vi "Panel.vi"(11 "ControlBindingPanel in":refnum<class "ControlBindingPanel.lvclass">) -> ()   [LabVIEW 2020, in "VolatusGUIEditor.lvlib" / "ControlBindingPanel.lvclass"]
uses:
  ControlBindingPanel.lvclass
  C:/dev/lv20CE/relink/lv-oopanel/OOPanel/Panel/Panel.lvclass
  lv-oopanel/OOPanel/Panel/Basic UI State.ctl
  ControlBindingPanel.lvclass/ControlBindingPanel.ctl
  Control Bind Data.ctl
  lv-tree-tools/Tree Map/Tree Map/Tree Map.lvclass
  lv-oopanel/OOPanel/Panel/Panel.lvclass
  lv-oopanel/OOPanel/OOPanel.lvlib
  VolatusGUIEditor.lvlib
panel:
  in  "Select":bool
  in  "Tree":string(tree)
  # "Selected element is not bound to a control type.\nSet the control type from the list below:"
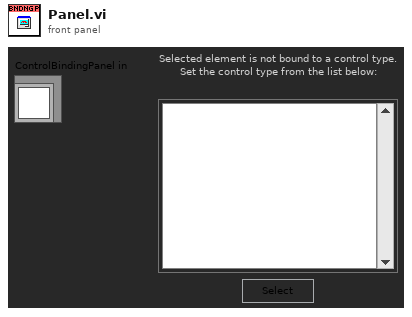
[diagram p1: front panel]
types:
  T1 = typedef "OOPanel.lvlib/Panel.lvclass/Basic UI State.ctl" = enum16{"Init", "Run", "Close"}
  T2 = enum8{"Enabled", "Disabled", "Disabled and Grayed Out"}
  T3 = typedef "VolatusGUIEditor.lvlib/Control Bind Data.ctl" = cluster{"Ctl Refnum":refnum<vi>, "Type Name":string}
  T4 = typedef "VolatusGUIEditor.lvlib/ControlBindingPanel.lvclass/Incoming Events.ctl" = cluster{"Update Control":refnum<user-event>, "Update Tree":refnum<user-event>}
  T5 = typedef "OOPanel.lvlib/Panel.lvclass/Panel Events.ctl" = cluster{"Visbility":refnum<user-event>, "Close":refnum<user-event>}
  T6 = typedef "OOPanel.lvlib/Visibility State.ctl" = enum16{"Idle", "Closed", "Hidden", "Visible", "Subpanel", "Hidden Subpanel"}
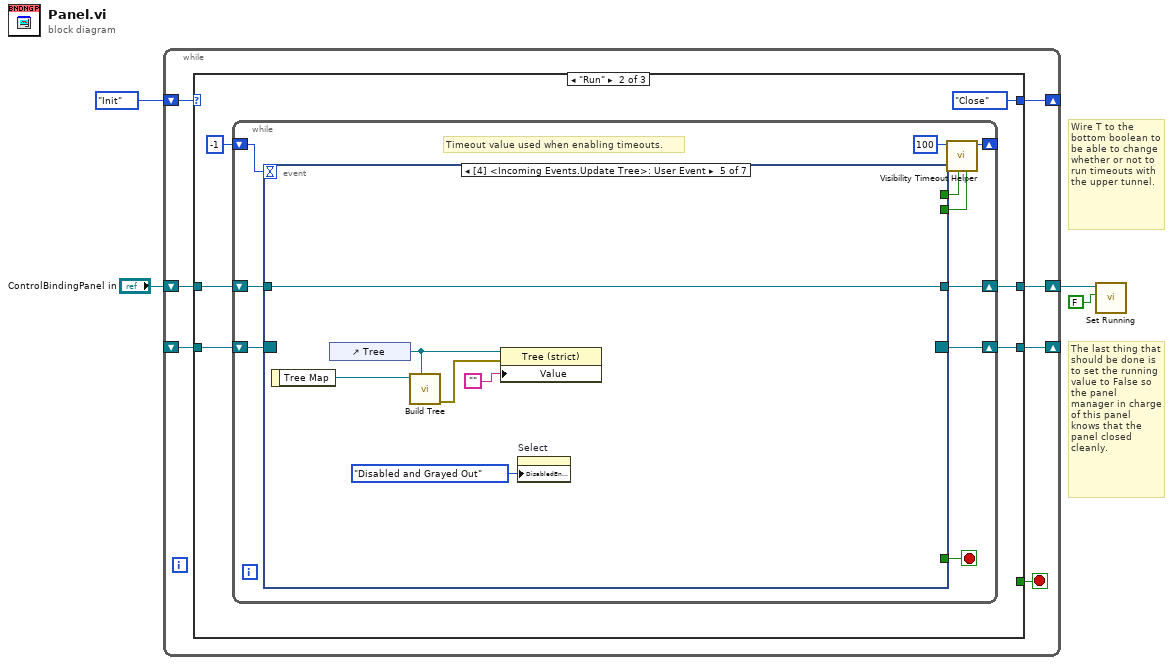
[diagram p0: block diagram]
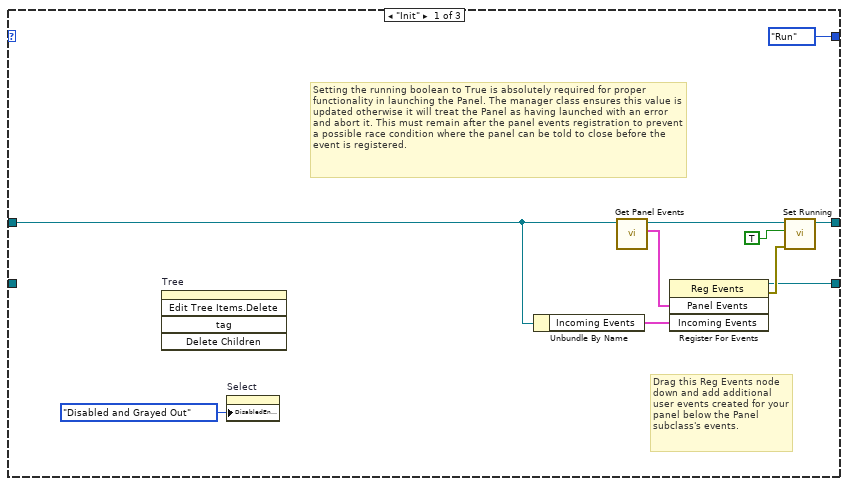
[diagram p2: hidden frame]
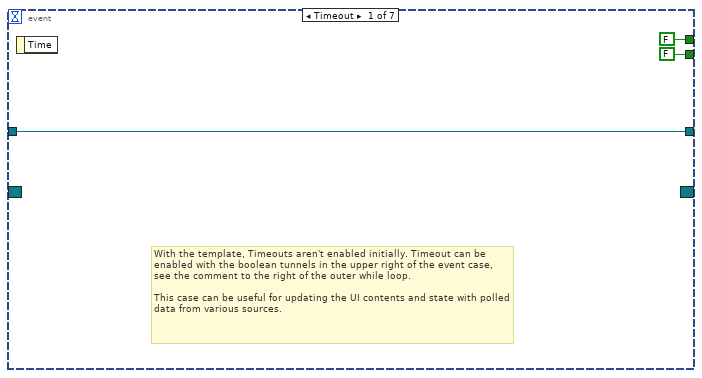
[diagram p3: hidden frame]
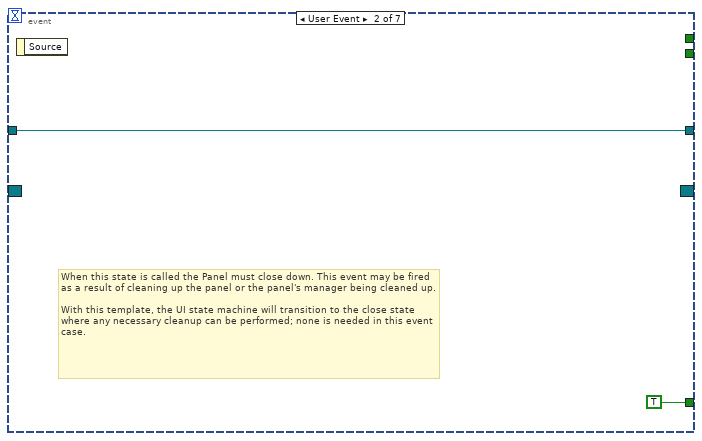
[diagram p4: hidden frame]
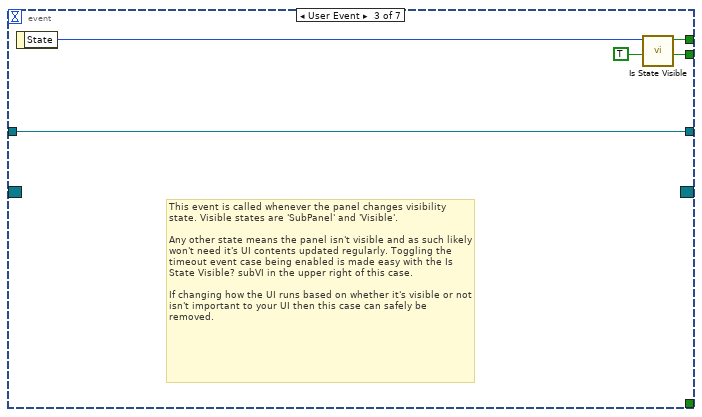
[diagram p5: hidden frame]
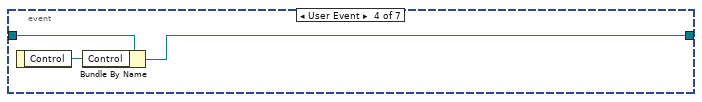
[diagram p6: hidden frame]
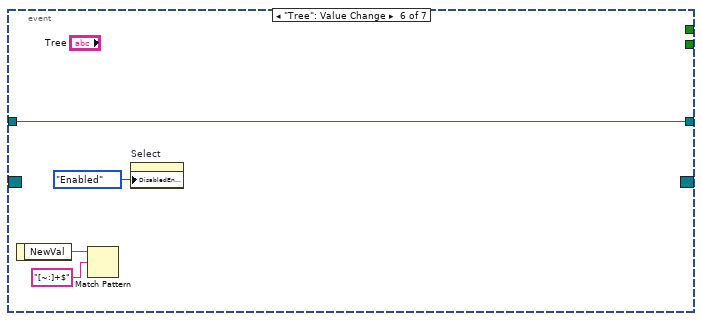
[diagram p7: hidden frame]
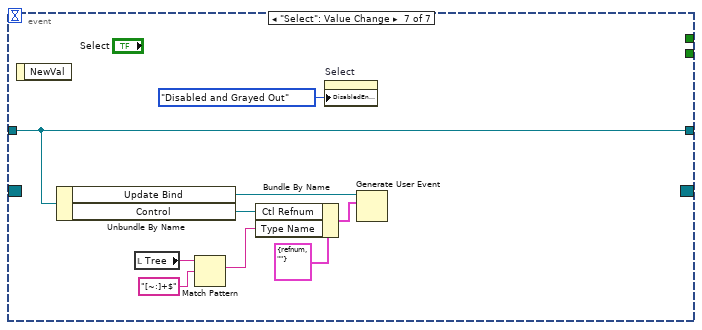
[diagram p8: hidden frame]
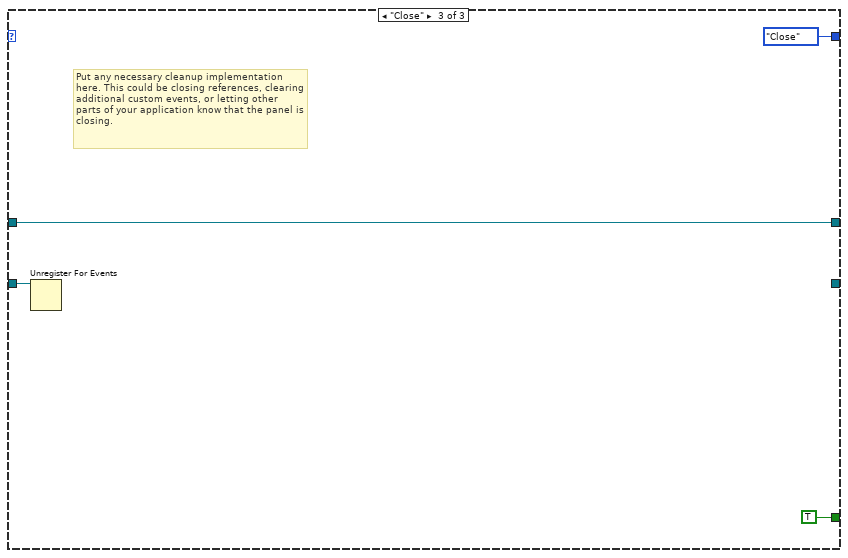
[diagram p9: hidden frame]
diagram:
  # "The last thing that should be done is to set the running value to False so the panel manager in charge of this panel knows that the panel closed cleanly."
  # "Wire T to the bottom boolean to be able to change whether or not to run timeouts with the upper tunnel."
  n1 = while {
    shift-right: [w10] -> _
    shift-left: _ -> [w11]
    shift-right: [w8] -> _
    shift-left: Basic_UI_State."Init" ("Basic UI State") -> [w9]
    shift-right: [w6] -> w4
    shift-left: "ControlBindingPanel in" -> [w5]
    stop <- w7 stop-if-true
    n2 = case shown="\"Run\"" w9 {
      tunnel: w11 -> [_ w27 w70]
      tunnel: [w18 w25 _] -> w10
      tunnel: [Basic_UI_State."Run" ("Basic UI State") Basic_UI_State."Close" ("Basic UI State") Basic_UI_State."Close" ("Basic UI State")] -> w8
      tunnel: [_ _ TRUE] -> w7
      tunnel: [w17 w22 w69] -> w6
      tunnel: w5 -> [w13 w23 w69]
      frame "Init" {
        # "Setting the running boolean to True is absolutely required for proper functionality in launching the Panel. The manager class ensures this value is updated otherwise it will treat the Panel as having launched with an error and abort it. This must remain after the panel events registration to prevent a possible race condition where the panel can be told to close before the event is registered."
        # "Drag this Reg Events node down and add additional user events created for your panel below the Panel subclass's events."
        n3 = invoke on="Tree" class="Tree (strict)" method="Edit Tree Items.Delete"() -> ()  [unwired: 5 in, 5 out]
        n4 = property on="Select" class="Bool"("DisabledEnum"=T2."Disabled and Grayed Out" ("Disabled")) -> ()  [unwired: 2 in, 2 out]
        n5 = Unbundle By Name(w13) -> ("Incoming Events"=w12:T4)
        n6 = call "Get Panel Events.vi"("Panel in"=w13) -> ("Panel Events"=w15:T5, "Panel out"=w16:refnum<class "ControlBindingPanel.lvclass">)  [unwired: 8 in, 1 out]
        n7 = register-events(w15, w12) -> (reference out=w18:refnum<event-registration>, error out=w20:errorcluster)  [unwired: 2 in]
        n8 = call "Set Running.vi"("error in (no error)"=w20, "Running"=TRUE, "Panel in"=w16) -> ("Panel out"=w17:refnum<class "ControlBindingPanel.lvclass">)  [unwired: 7 in, 1 out]
      }
      frame "Run" {
        n9 = while {
          shift-right: [w33] -> w25
          shift-left: w27 -> [w34]
          shift-right: [w36] -> _
          shift-left: -1 ("Timeout") -> [w35]
          shift-right: [w28] -> w22
          shift-left: w23 -> [w29]
          stop <- w30 stop-if-true
          # "Timeout value used when enabling timeouts."
          n10 = event shown="[4] <Incoming Events.Update Tree>: User Event" {
            selector: w34 -> [_ _ _ _ _ _ _]
            dyn-events: [_ _ _ _ _ _ _] -> w33
            timeout: w35 -> [_ _ _ _ _ _ _]
            tunnel: [FALSE _ w45 _ _ _ _] -> w32
            tunnel: [FALSE _ TRUE _ _ _ _] -> w31
            tunnel: [_ TRUE _ _ _ _ _] -> w30
            tunnel: w29 -> [w38 w41 w43 w49 w55 w59 w66]
            tunnel: [w38 w41 w43 w48 w55 w59 w66] -> w28
            event Timeout {
              # "With the template, Timeouts aren't enabled initially. Timeout can be enabled with the boolean tunnels in the upper right of the event case, see the comment to the right of the outer while loop.\n\nThis case can be useful for updating the UI contents and state with polled data from various sources."
              n11 = event-data() -> ()  [unwired: 1 in, 1 out]
            }
            event User Event {
              # "When this state is called the Panel must close down. This event may be fired as a result of cleaning up the panel or the panel's manager being cleaned up.\n\nWith this template, the UI state machine will transition to the close state where any necessary cleanup can be performed; none is needed in this event case."
              n12 = event-data() -> ()  [unwired: 1 in, 1 out]
            }
            event User Event {
              # "This event is called whenever the panel changes visibility state. Visible states are 'SubPanel' and 'Visible'.\n\nAny other state means the panel isn't visible and as such likely won't need it's UI contents updated regularly. Toggling the timeout event case being enabled is made easy with the Is State Visible? subVI in the upper right of this case.\n\nIf changing how the UI runs based on whether it's visible or not isn't important to your UI then this case can safely be removed."
              n13 = event-data() -> ("State"=w46:T6)  [unwired: 1 in]
              n14 = call "Is State Visible.vi"("Visibility"=w46) -> ("Visible"=w45:bool)  [unwired: 10 in]
            }
            event User Event {
              n15 = event-data() -> ("Control"=w47:refnum<vi>)  [unwired: 1 in]
              n16 = Bundle By Name(cluster=w49, "Control"=w47) -> (w48:refnum<class "ControlBindingPanel.lvclass">)
            }
            event User Event {
              n17 = event-data() -> ("Tree Map"=w54:refnum<class "Tree Map.lvclass">)  [unwired: 1 in]
              n18 = control-ref of="Tree"() -> (w53:refnum<vi>)
              n19 = call "Build Tree.vi"("Tree"=w53, "Tree Map in"=w54) -> ("error out"=w52:errorcluster)  [unwired: 8 in, 1 out]
              n20 = property class="Tree (strict)"(reference=w53, error in=w52, "Value"="") -> ()  [unwired: 2 out]
              n21 = property on="Select" class="Bool"("DisabledEnum"=T2."Disabled and Grayed Out" ("Disabled")) -> ()  [unwired: 2 in, 2 out]
            }
            event "Tree": Value Change {
              n22 = event-data() -> ("NewVal"=w58:string)  [unwired: 1 in]
              n23 = Match Pattern(string=w58, regular expression="[~:]+$") -> ()  [unwired: 1 in, 4 out]
              n24 = property on="Select" class="Bool"("DisabledEnum"=T2."Enabled" ("Disabled")) -> ()  [unwired: 2 in, 2 out]
            }
            event "Select": Value Change {
              n25 = event-data() -> ()  [unwired: 1 in, 1 out]
              n26 = Unbundle By Name(w66) -> ("Update Bind"=w65:refnum<user-event>, "Control"=w62:refnum<vi>)
              n27 = local read "Tree"() -> (w67:string)
              n28 = Match Pattern(string=w67, regular expression="[~:]+$") -> (match substring=w61:string)  [unwired: 1 in, 3 out]
              n29 = Bundle By Name(cluster=T3 {"Ctl Refnum"=refnum, "Type Name"=""} ("event data"), "Ctl Refnum"=w62, "Type Name"=w61) -> (w63:T3)
              n30 = property on="Select" class="Bool"("DisabledEnum"=T2."Disabled and Grayed Out" ("Disabled")) -> ()  [unwired: 2 in, 2 out]
              n31 = Generate User Event(user event=w65, event data cluster=w63) -> ()  [unwired: 2 in, 2 out]
            }
          }
          n32 = call "Visibility Timeout Helper.vi"("Update?"=w31, "Use Timeout?"=w32, "Visible Timeout mS"=100) -> ("Timeout"=w36:i32)  [unwired: 8 in]
        }
      }
      frame "Close" {
        # "Put any necessary cleanup implementation here. This could be closing references, clearing additional custom events, or letting other parts of your application know that the panel is closing."
        n33 = Unregister For Events(event registration refnum=w70) -> ()  [unwired: 1 in, 1 out]
      }
    }
  }
  n34 = call "Set Running.vi"("Running"=FALSE, "Panel in"=w4) -> ()  [unwired: 8 in, 2 out]
